vi "cursor test.vi"() -> ()   [LabVIEW 2019]
uses:
  <vilib>/Utility/miscctls.llb/LVCursorListTypeDef.ctl
  <vilib>/gmath/NI_Gmath.lvlib
panel:
  in  "Delete Cursor":bool
  in  "Graph Points":i32=50
  in  "Interpolation Method":i32(ring)=1 items=["nearest", "linear", "spline", "cubic Hermite", "Lagrange"]
  in  "Add Cursor":bool
  out "XY Graph":cluster{dbl[], dbl[]}(graph)
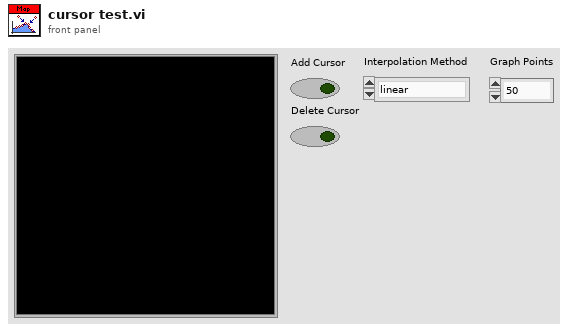
[diagram p1: front panel]
types:
  T1 = typedef "LVCursorListTypeDef.ctl" = cluster{"Name":string, "Color":u32, "Style":u8, "Point Style":u8, "Name Visible":bool, "Allow Drag":bool, "Cursor Mode":u32, "Plot":i32, "Index":i32, "Position":cluster{"X":dbl, "Y":dbl}, "X Scale":u32, "Y Scale":u32, "Watch Plots":i32[], "Watch All Plots":bool, "Plot Area":i32, "Label Offset":cluster{"X":dbl, "Y":dbl}}[]
  T2 = cluster{"Name":string, "Color":u32, "Style":u8, "Point Style":u8, "Name Visible":bool, "Allow Drag":bool, "Cursor Mode":u32, "Plot":i32, "Index":i32, "Position":cluster{"X":dbl, "Y":dbl}, "X Scale":u32, "Y Scale":u32, "Watch Plots":i32[], "Watch All Plots":bool, "Plot Area":i32, "Label Offset":cluster{"X":dbl, "Y":dbl}}
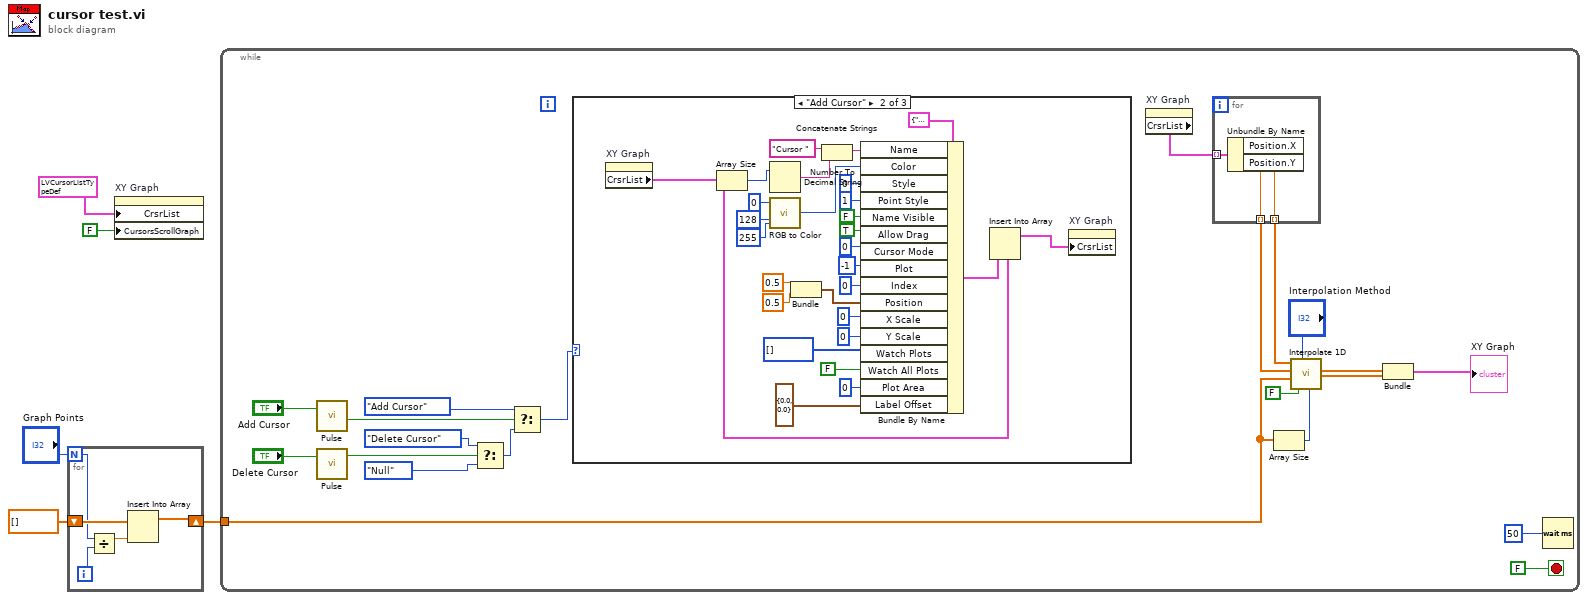
[diagram p0: block diagram]
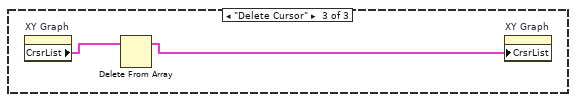
[diagram p3: hidden frame]
diagram:
  n1 = for {
    N: "Graph Points" -> [w7]
    shift-right: [w9] -> w4
    shift-left: dbl[] [] -> [w8]
    i -> [w6]
    n2 = Divide(x=w6, y=w7) -> (x/y=w10:dbl)
    n3 = Insert Into Array(array=w8, new element=w10) -> (w9:dbl[])  [unwired: 1 in]
  }
  n4 = property on="XY Graph" class="XYGraph (strict)"("CrsrList"=T1 [{"Name"="Cursor 0", "Color"=33023, "Style"=0, "Point Style"=1, "Name Visible"=FALSE, "Allow Drag"=TRUE, "Cursor Mode"=0, "Plot"=-1, "Index"=0, "Position"={"X"=0.5, "Y"=0.5}, "X Scale"=0, "Y Scale"=0, "Watch Plots"=[], "Watch All Plots"=FALSE, "Plot Area"=0, "Label Offset"={"X"=0.0, "Y"=0.0}}] ("Cursor List"), "CursorsScrollGraph"=FALSE ("Cursors Scroll Graph")) -> ()  [unwired: 2 in, 2 out]
  n5 = while {
    tunnel: w4 -> [w20]
    stop <- FALSE stop-if-true
    n6 = call "Pulse.vi"("Input"="Add Cursor") -> ("Output"=w16:bool)  [unwired: 10 in]
    n7 = call "Pulse.vi"("Input"="Delete Cursor") -> ("Output"=w17:bool)  [unwired: 10 in]
    n8 = Select(t=enum16{"Null", "Add Cursor", "Delete Cursor"}."Delete Cursor", s=w17, f=enum16{"Null", "Add Cursor", "Delete Cursor"}."Null") -> (s? t:f=w13:enum16{"Null", "Add Cursor", "Delete Cursor"})
    n9 = Select(t=enum16{"Null", "Add Cursor", "Delete Cursor"}."Add Cursor", s=w16, f=w13) -> (s? t:f=w11:enum16{"Null", "Add Cursor", "Delete Cursor"})
    n10 = case shown="\"Add Cursor\"" w11 {
      frame "Null", Default {
      }
      frame "Add Cursor" {
        n11 = property on="XY Graph" class="XYGraph (strict)"() -> ("CrsrList"=w36:T1)  [unwired: 2 in, 2 out]
        n12 = Array Size(array=w36) -> (size(s)=w39:i32)
        n13 = Number To Decimal String(number=w39) -> (decimal integer string=w59:string)  [unwired: 1 in]
        n14 = call <vilib>:"RGB to Color.vi"("B"=u8 255, "G"=u8 128, "R"=u8 0) -> ("Color"=w57:u32)
        n15 = Bundle(0.5, 0.5) -> (w40:cluster{dbl, dbl})  [unwired: 1 in]
        n16 = Concatenate Strings("Cursor ", w59) -> (w58:string)
        n17 = Bundle By Name(cluster=T2 {"Name"="", "Color"=33023, "Style"=0, "Point Style"=0, "Name Visible"=FALSE, "Allow Drag"=FALSE, "Cursor Mode"=0, "Plot"=0, "Index"=0, "Position"={"X"=0.0, "Y"=0.0}, "X Scale"=0, "Y Scale"=0, "Watch Plots"=[], "Watch All Plots"=FALSE, "Plot Area"=0, "Label Offset"={"X"=0.0, "Y"=0.0}} ("Cursor List"), "Name"=w58, "Color"=w57, "Style"=u8 0, "Point Style"=u8 1, "Name Visible"=FALSE, "Allow Drag"=TRUE, "Cursor Mode"=u32 0, "Plot"=-1, "Index"=0, "Position"=w40, "X Scale"=u32 0, "Y Scale"=u32 0, "Watch Plots"=i32[] [], "Watch All Plots"=FALSE, "Plot Area"=0, "Label Offset"=cluster{"X":dbl, "Y":dbl} {"X"=0.0, "Y"=0.0}) -> (w62:T2)
        n18 = Insert Into Array(array=w36, new element=w62) -> (w61:T1)  [unwired: 1 in]
        n19 = property on="XY Graph" class="XYGraph (strict)"("CrsrList"=w61) -> ()  [unwired: 2 in, 2 out]
      }
      frame "Delete Cursor" {
        n20 = property on="XY Graph" class="XYGraph (strict)"() -> ("CrsrList"=w64:T1)  [unwired: 2 in, 2 out]
        n21 = Delete From Array(array=w64) -> (array with subset deleted=w63:T1)  [unwired: 2 in, 1 out]
        n22 = property on="XY Graph" class="XYGraph (strict)"("CrsrList"=w63) -> ()  [unwired: 2 in, 2 out]
      }
    }
    n23 = property on="XY Graph" class="XYGraph (strict)"() -> ("CrsrList"=w29:T1)  [unwired: 2 in, 2 out]
    n24 = for {
      tunnel: w29 -> [w34] mode=indexing
      tunnel: [w33] -> w28 mode=indexing
      tunnel: [w32] -> w27 mode=indexing
      n25 = Unbundle By Name(w34) -> ("Position.X"=w33:dbl, "Position.Y"=w32:dbl)
    }
    n26 = Array Size(array=w20) -> (size(s)=w25:i32)
    n27 = call <vilib>:"Interpolate 1D.vi"("ntimes"=w25, "method"="Interpolation Method", "X is monotonic"=FALSE, "xi"=w20, "X"=w28, "Y"=w27) -> ("xi used"=w24:dbl[], "yi"=w23:dbl[])  [unwired: 3 in, 1 out]
    n28 = Bundle("xi used"=w24, "yi"=w23) -> (→"XY Graph":cluster{"xi used":dbl[], "yi":dbl[]})  [unwired: 1 in]
    n29 = Wait (ms)(milliseconds to wait=u32 50) -> ()  [unwired: 1 out]
  }
